vi "Config Measure Phase.vi"(0 "VISA resource name":refnum<visa-resource-name>, 5 "Phase (0: 180 Lead/Lag)":u16(ring) items=["180 Lead/Lag", "360 degrees"], 11 "error in (no error)":errorcluster) -> (4 "VISA resource name out":refnum<visa-resource-name>, 15 "error out":errorcluster)   [LabVIEW 2013, in "Yokogawa.lvlib" / "Yokogawa PZ4000.lvlib"]
doc: "This VI sends the Measure Phase group command to the PZ4000 series."
uses:
  Yokogawa PZ4000.lvlib
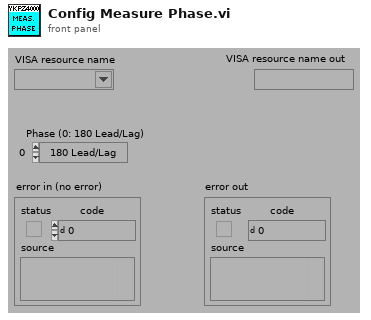
[diagram p1: front panel]
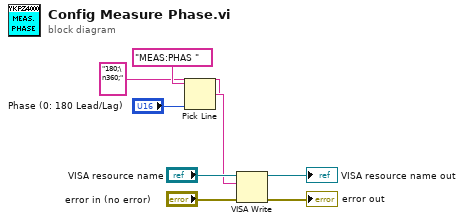
[diagram p0: block diagram]
diagram:
  n1 = Pick Line(string ("")="MEAS:PHAS ", multi-line string="180;\n360;", line index="Phase (0: 180 Lead/Lag)") -> (output string=w2:string)
  n2 = VISA Write(VISA resource name="VISA resource name", write buffer=w2, error in (no error)="error in (no error)") -> (VISA resource name out=→"VISA resource name out":refnum<visa-resource-name>, error out=→"error out":errorcluster)  [unwired: 1 out]
